vi "Assign Bitmap.vi"(8 "error in (no error)":errorcluster, 10 "bitmap":u8[][](array[numeric]), 11 "ElectrodeGrid in":refnum<class "ElectrodeGrid.lvclass">) -> (0 "error out":errorcluster, 3 "ElectrodeGrid out":refnum<class "ElectrodeGrid.lvclass">)   [LabVIEW 2017, in "ElectrodeGrid.lvclass"]
uses:
  ElectrodeGrid.lvclass
  ElectrodeGrid.lvclass/ElectrodeGrid.ctl
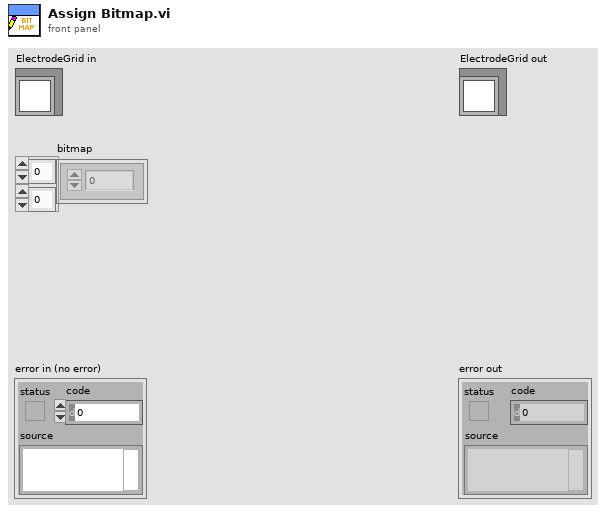
[diagram p1: front panel]
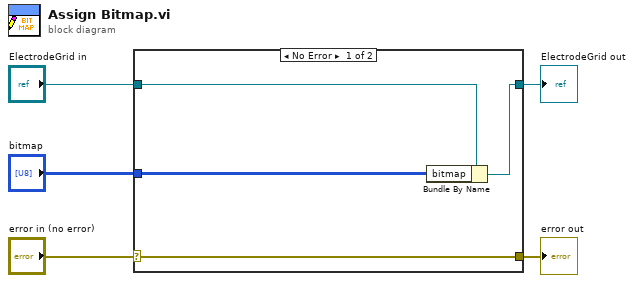
[diagram p0: block diagram]
diagram:
  n1 = case shown="No Error" "error in (no error)" {
    selector: "error in (no error)" -> [w9 w10]
    tunnel: [w9 w10] -> w4
    tunnel: [w7 w11] -> w2
    tunnel: "ElectrodeGrid in" -> [w8 w11]
    tunnel: "bitmap" -> [w6 _]
    frame No Error {
      n2 = Bundle By Name(cluster=w8, "bitmap"=w6) -> (w7:refnum<class "ElectrodeGrid.lvclass">)
    }
    frame Error {
    }
  }
  "error out" <- w4
  "ElectrodeGrid out" <- w2
